vi "Day 20-Calculate Lookup Index.vi"(9 "Left of Subgrid":i32, 10 "Top of Subgrid":i32, 11 "Image in":bool[][](array[boolean])) -> (3 "Lookup Index":u32)   [LabVIEW 2021]
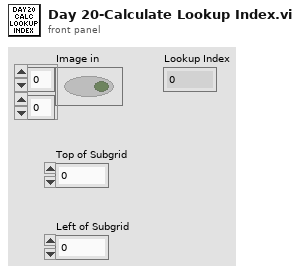
[diagram p1: front panel]
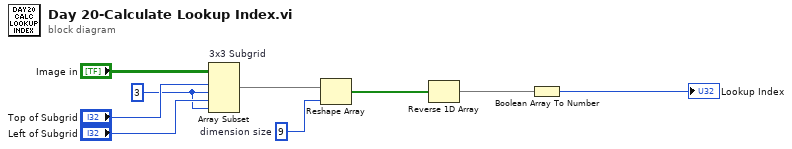
[diagram p0: block diagram]
diagram:
  w4 = 9  # dimension size
  w2 = 3 ("length")
  n1 = Array Subset "3x3 Subgrid"(array="Image in", index (row)="Top of Subgrid", length (row)=w2, index (col)="Left of Subgrid", length (col)=w2) -> (w3:bool[][])
  n2 = Reshape Array "Reshape Array"(w3, w4) -> (w5:bool[])
  n3 = Reverse 1D Array(array=w5) -> (reversed array=w9:bool[])
  n4 = Boolean Array To Number(Boolean array=w9) -> (number=→"Lookup Index":u32)
